vi "Laser.vi"(8 "error IO":errorcluster) -> (0 "error Out":errorcluster, 3 "Laser1":dbl)   [LabVIEW 2019]
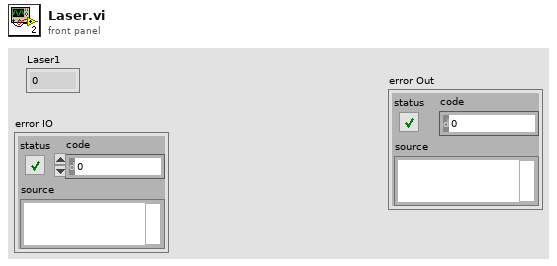
[diagram p1: front panel]
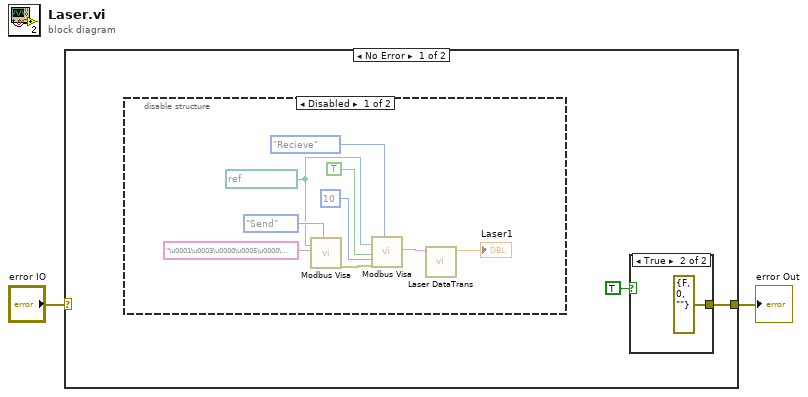
[diagram p0: block diagram]
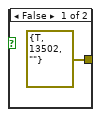
[diagram p3: hidden frame]
diagram:
  n1 = case shown="No Error" "error IO" {
    selector: "error IO" -> [_ w16]
    tunnel: [w4 w16] -> w1
    frame No Error {
      n2 = disable-structure shown="Disabled" {
        frame Disabled {
          w5 = refnum<visa-resource-name> "COM11" ("VISA resource name")
          n3 = call "Modbus Visa.vi"("VISA resource name"=w5, "Cmd"="\u0001\u0003\u0000\u0005\u0000\u0002Ô\n", "VisaAction"=enum16{"Open", "Send", "Recieve", "Close"}."Send") -> ("error out"=w9:errorcluster)  [unwired: 15 in, 1 out]
          n4 = call "Modbus Visa.vi"("VISA resource name"=w5, "TimeOut"=TRUE, "Time(0.1)"=u32 10, "error in (no error)"=w9, "VisaAction"=enum16{"Open", "Send", "Recieve", "Close"}."Recieve") -> ("read string"=w8:string)  [unwired: 13 in, 1 out]
          n5 = call "Laser DataTrans.vi"("Strin"=w8) -> ("Read"=→"Laser1":dbl)  [unwired: 10 in]
        }
        frame Enabled {
        }
      }
      n6 = case shown="True" TRUE {
        tunnel: [errorcluster {"status"=TRUE, "code"=13502, "source"=""} ("error constant") errorcluster {"status"=FALSE, "code"=0, "source"=""} ("error constant")] -> w4
        frame False {
        }
        frame True {
        }
      }
    }
    frame Error {
    }
  }
  "error Out" <- w1
